vi "Add Version and Language JSON Entries.vi"(8 "error in":errorcluster, 10 "JSON in":string, 11 "nats connection in":T1) -> (0 "error out":errorcluster, 2 "JSON out":string, 3 "nats connection out":T1)   [LabVIEW 2013, in "NATS Core.lvlib"]
doc: "Adds \"version\", \"headers\", and \"lang\" entries to the JSON string if they are not already present."
uses:
  NATS Core.lvlib
  Controls/nats connection.ctl
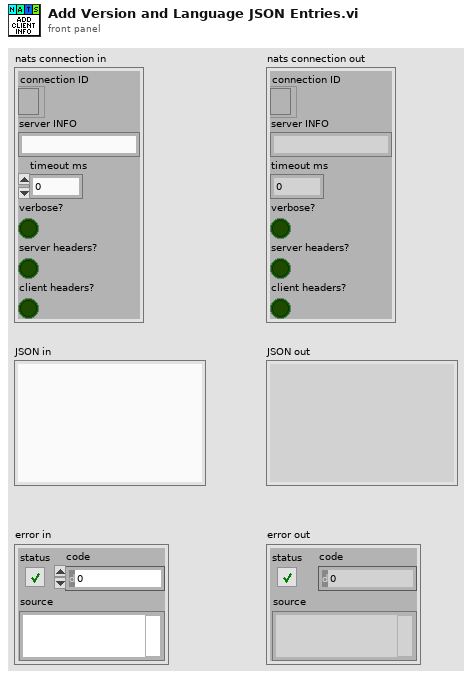
[diagram p1: front panel]
types:
  T1 = typedef "NATS Core.lvlib/nats connection.ctl" = cluster{"connection ID":refnum<k5>, "server INFO":string, "timeout ms":i32, "verbose?":bool, "server headers?":bool, "client headers?":bool}
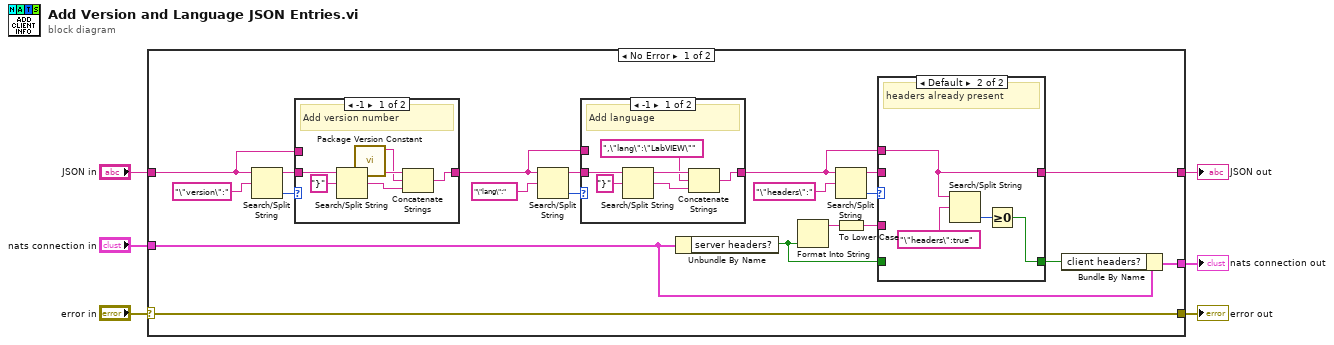
[diagram p0: block diagram]
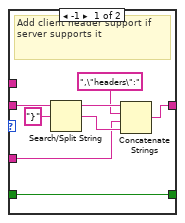
[diagram p4: hidden frame]
diagram:
  n1 = case shown="No Error" "error in" {
    selector: "error in" -> [w20 w55]
    tunnel: [w13 w54] -> w6
    tunnel: "JSON in" -> [w19 w54]
    tunnel: [w20 w55] -> w3
    tunnel: "nats connection in" -> [w10 w53]
    tunnel: [w7 w53] -> w1
    frame No Error {
      n2 = Search/Split String(string=w19, search string/char (-)="\"version\":") -> (substring before match=w23:string, offset of match=w22:i32)  [unwired: 1 in, 1 out]
      n3 = case shown="-1" w22 {
        tunnel: w23 -> [w39 _]
        tunnel: [w34 w40] -> w18
        tunnel: w19 -> [_ w40]
        frame -1 {
          # "Add version number"
          n4 = Search/Split String(string=w39, search string/char (-)="}") -> (substring before match=w37:string, match + rest of string=w35:string)  [unwired: 1 in, 1 out]
          n5 = call "Package Version Constant.vi"() -> ("package_version"=w36:string)  [unwired: 11 in]
          n6 = Concatenate Strings(w37, w36, w35) -> (w34:string)
        }
        frame Default {
          # "version already present"
        }
      }
      n7 = Search/Split String(string=w18, search string/char (-)="\"lang\":") -> (substring before match=w24:string, offset of match=w25:i32)  [unwired: 1 in, 1 out]
      n8 = case shown="-1" w25 {
        tunnel: w24 -> [w32 _]
        tunnel: [w28 w33] -> w14
        tunnel: w18 -> [_ w33]
        frame -1 {
          # "Add language"
          n9 = Search/Split String(string=w32, search string/char (-)="}") -> (substring before match=w30:string, match + rest of string=w29:string)  [unwired: 1 in, 1 out]
          n10 = Concatenate Strings(w30, ",\"lang\":\"LabVIEW\"" ("string"), w29) -> (w28:string)
        }
        frame Default {
          # "lang already present"
        }
      }
      n11 = Unbundle By Name(w10) -> ("server headers?"=w8:bool)
      n12 = Format Into String(w8) -> (resulting string=w12:string)  [unwired: 3 in, 1 out]
      n13 = Search/Split String(string=w14, search string/char (-)="\"headers\":") -> (substring before match=w17:string, offset of match=w16:i32)  [unwired: 1 in, 1 out]
      n14 = To Lower Case(string=w12) -> (all lower case string=w11:string)
      n15 = case shown="Default" w16 {
        tunnel: w17 -> [w48 _]
        tunnel: [w45 w49] -> w13
        tunnel: w14 -> [_ w49]
        tunnel: w11 -> [w42 _]
        tunnel: [w41 w50] -> w9
        tunnel: w8 -> [w41 _]
        frame -1 {
          # "Add client header support if server supports it"
          n16 = Search/Split String(string=w48, search string/char (-)="}") -> (substring before match=w46:string, match + rest of string=w43:string)  [unwired: 1 in, 1 out]
          n17 = Concatenate Strings(w46, ",\"headers\":" ("string"), w42, w43) -> (w45:string)
        }
        frame Default {
          # "headers already present"
          n18 = Search/Split String(string=w49, search string/char (-)="\"headers\":true") -> (offset of match=w51:i32)  [unwired: 1 in, 2 out]
          n19 = Greater Or Equal To 0?(x=w51) -> (x >= 0?=w50:bool)
        }
      }
      n20 = Bundle By Name(cluster=w10, "client headers?"=w9) -> (w7:T1)
    }
    frame Error {
    }
  }
  "JSON out" <- w6
  "error out" <- w3
  "nats connection out" <- w1
